vi "Main Page.vi"(8 "error in (no error)":errorcluster, 11 "Node Ptr":T1 format="%.0x") -> (0 "error out":errorcluster)   [LabVIEW 2023, in "J1939 Addon System Explorer.lvlib"]
uses:
  J1939 Addon System Explorer.lvlib
  <vilib>/NI VeriStand/Custom Device API/Custom Device Item Ref.ctl
  <vilib>/NI/NI VeriStand Hardware Resource Discovery/_Types/Filter Type.ctl
  <vilib>/NI VeriStand/Custom Device API/Custom Device File Dependency.ctl
  <vilib>/NI VeriStand/Custom Device API/Path Specification.ctl
  <vilib>/NI VeriStand/Custom Device API/Path Type.ctl
  <vilib>/NI VeriStand/Custom Device API/Custom Device Supported Target.ctl
  Addon Shared/SubVIs/Constants.vi
  <vilib>/NI VeriStand/Custom Device API/Get Item Property (Boolean).vi
  <vilib>/NI VeriStand/Custom Device API/Set Item Property (Boolean).vi
  <vilib>/NI VeriStand/Custom Device API/Set Item Property (String).vi
  <vilib>/NI VeriStand/Custom Device API/Set Item Property (Path).vi
  <vilib>/NI VeriStand/Custom Device API/Get Item Property (String).vi
  <vilib>/NI VeriStand/Custom Device API/Get Item Property (Path).vi
  <vilib>/NI VeriStand/Custom Device API/Custom Device API.lvlib
  Addon Shared/J1939 Addon Shared.lvlib
  <vilib>/NI/NI VeriStand Hardware Resource Discovery/NIVS Hardware Discovery.lvlib
panel:
  out "Version":string
  in  "RIO Browse":bool
  in  "CAN Browse":bool
  in  "Outcoming Decimation":u32=100
  in  "Incoming Decimation":u32=100
  in  "J1939 Settings 3":cluster{"Section Name":string}={"Section Name"="NI 986x Settings"}
  in  "J1939 Database Settings":cluster{"Section Name":string}={"Section Name"="J1939 Database Settings"}
  in  "RIO Device":string
  in  "Bitfile Path":path
  in  "Enable Bitfile":bool
  in  "Termination":enum16{"Off", "On"}(ring)
  in  "SHDocVw.IWebBrowser2":refnum<k7>(container)
  in  "NI 986x Settings":cluster{"Section Name":string}={"Section Name"="CAN Settings"}
  in  "CAN Port":string
  in  "Baud rate [Bd]":u32 format="%.0p"
  out "XNET Cluster":refnum<k21>
  out "XNET Database":refnum<k21>
  in  "Name":string
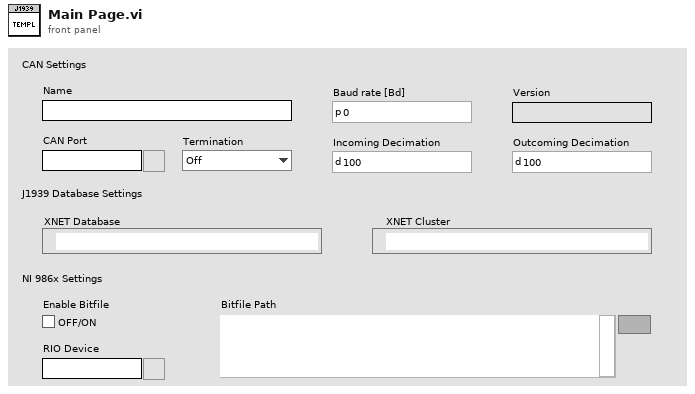
[diagram p1: front panel]
types:
  T1 = typedef "Custom Device API.lvlib/Custom Device Item Ref.ctl" = u64
  T2 = typedef "Custom Device API.lvlib/Custom Device Item Info.ctl" = cluster{"Name":string, "Is Channel":bool, "GUID":string, "Is Waveform":bool}
  T3 = typedef "J1939 Addon Shared.lvlib/XNET Settings.ctl" = cluster{"Database":refnum<k21>, "Cluster":refnum<k21>, "Port":string, "Baud rate [Bd]":u32, "Termination":u32, "Incoming Decimation":u32, "Outgoing Decimation":u32}
  T4 = typedef "NIVS Hardware Discovery.lvlib/Filter Type.ctl" = enum16{"Device Category", "Product Name", "Ethernet", "XNET", "VISA", "FPGA", "EtherCAT Master", "DAQmx", "GPIB", "Serial"}
  T5 = typedef "Custom Device API.lvlib/Custom Device File Dependency.ctl" = cluster{"Source":T6, "RT Destination":path, "ForceDownload?":bool, "SupportedTarget":T8, "Version":string}
  T6 = typedef "Custom Device API.lvlib/Path Specification.ctl" = cluster{"Path":path, "Type":T7}
  T7 = typedef "Custom Device API.lvlib/Path Type.ctl" = enum16{"Absolute", "To Base", "To Common Data Dir", "To Application Data Dir"}
  T8 = typedef "Custom Device API.lvlib/Custom Device Supported Target.ctl" = enum16{"All", "PharLap", "VxWorks", "Windows", "Linux_32_ARM", "Linux_x64", "PharLap & Windows", "PharLap & VxWorks", "VxWorks & Windows"}
  T9 = typedef "Custom Device API.lvlib/Custom Device Commands.ctl" = enum16{"Default", "Item renamed", "Shutdown", "Dynamic button pressed"}
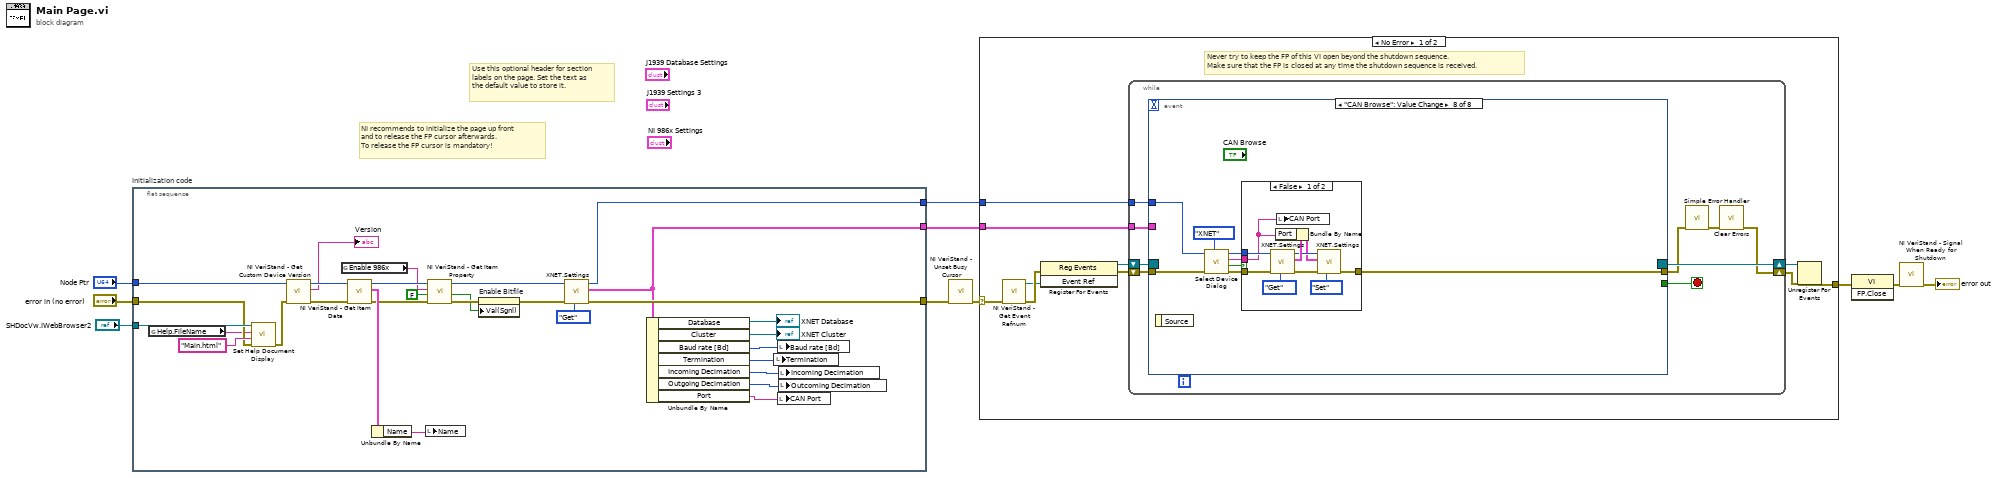
[diagram p0: block diagram]
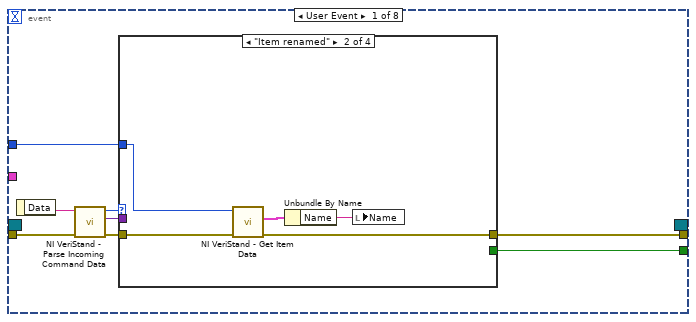
[diagram p2: hidden frame]
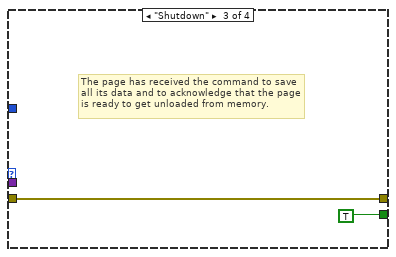
[diagram p4: hidden frame]
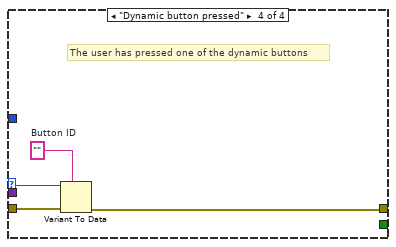
[diagram p5: hidden frame]
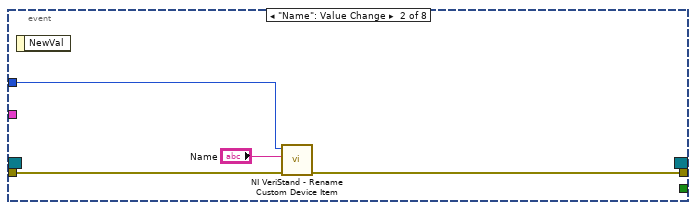
[diagram p6: hidden frame]
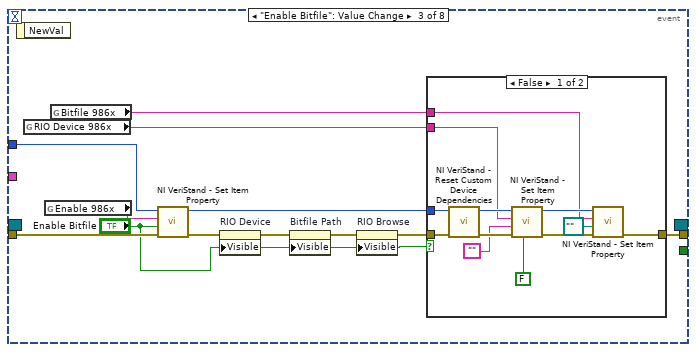
[diagram p7: hidden frame]
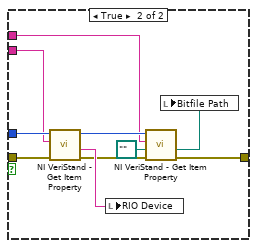
[diagram p8: hidden frame]
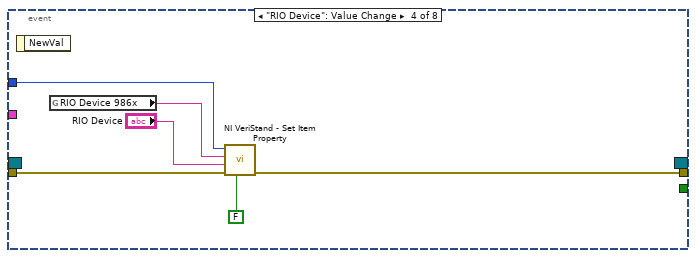
[diagram p9: hidden frame]
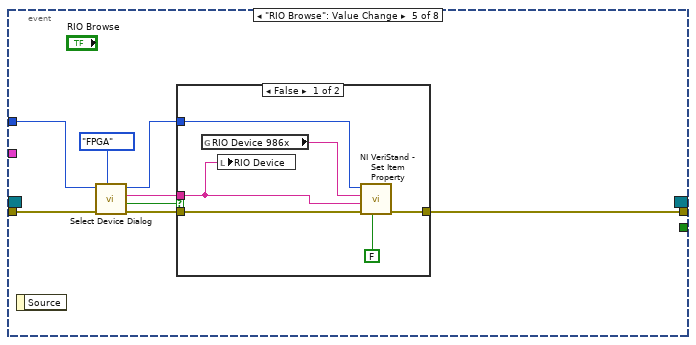
[diagram p10: hidden frame]
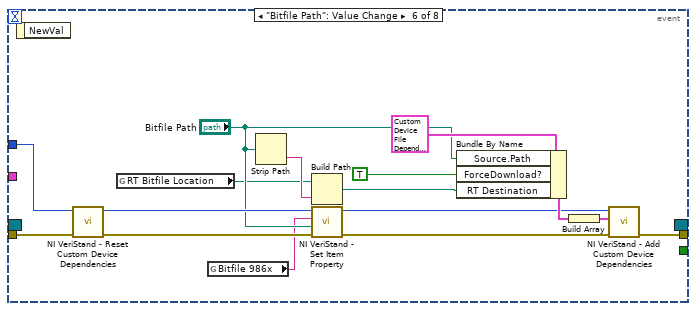
[diagram p12: hidden frame]
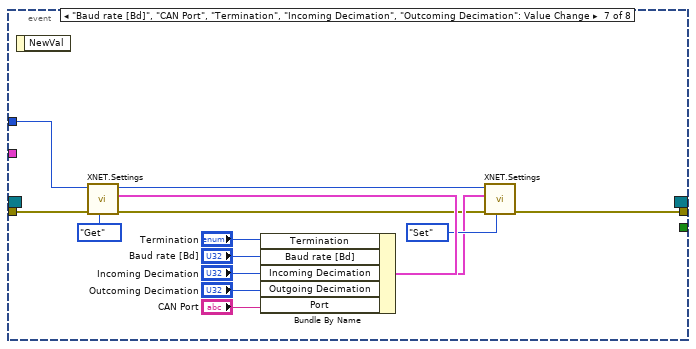
[diagram p13: hidden frame]
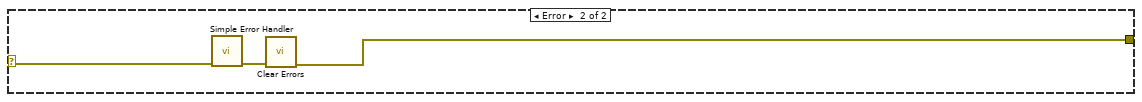
[diagram p15: hidden frame]
diagram:
  # "Use this optional header for section labels on the page. Set the text as the default value to store it."
  # "NI recommends to initialize the page up front\nand to release the FP cursor afterwards.\nTo release the FP cursor is mandatory!"
  n1 = flat-sequence "Initialization code" {
    tunnel: "error in (no error)" -> [w34]
    tunnel: "Node Ptr" -> [w13]
    tunnel: [w21] -> w6
    tunnel: [w38] -> w3
    tunnel: "SHDocVw.IWebBrowser2" -> [w35]
    tunnel: [w20] -> w1
    frame #0 {
      n2 = global read "Constants.vi" "Help.FileName"() -> (w11:string)
      n3 = call "Set Help Document Display.vi"("error in (no error)"=w34, "HTML File"="Main.html", "Main CHM File"=w11, "SHDocVw.IWebBrowser2"=w35) -> ("error out"=w16:errorcluster)  [unwired: 7 in]
      n4 = call <vilib>:"NI VeriStand - Get Custom Device Version.vi"("error in (no error)"=w16, "Device Ref in"=w13) -> ("error out"=w15:errorcluster, "Value"=→"Version":string, "Device Ref out"=w14:T1)  [unwired: 7 in]
      n5 = global read "Constants.vi" "Enable 986x"() -> (w29:string)
      n6 = call <vilib>:"NI VeriStand - Get Item Data.vi"("error in (no error)"=w15, "Item Ref in"=w14) -> ("error out"=w17:errorcluster, "Item Info"=w40:T2, "Item Ref out"=w31:T1)  [unwired: 7 out]
      n7 = Unbundle By Name(w40) -> ("Name"=w39:string)
      n8 = local write "Name"(w39) -> ()
      n9 = call-poly <vilib>:"NI VeriStand - Get Item Property.vi"("error in (no error)"=w17, "Default Value"=FALSE, "Property Name"=w29, "Item Ref in"=w31) -> ("error out"=w28:errorcluster, "Value"=w26:bool, "Item Ref out"=w30:T1)  [unwired: 4 in, 1 out]
      n10 = property on="Enable Bitfile" class="Bool (strict)"(error in=w28, "Val(Sgnl)"=w26) -> (error out=w27:errorcluster)  [unwired: 1 in, 1 out]
      n11 = call "XNET.Settings.vi"("Action"=enum8{"Get", "Set"}."Get", "error in (no error)"=w27, "Parent Ref in"=w30) -> ("error out"=w21:errorcluster, "J1939 XNET Settings"=w20:T3, "Item Ref out"=w38:T1)  [unwired: 6 in]
      n12 = Unbundle By Name(w20) -> ("Database"=→"XNET Database":refnum<k21>, "Cluster"=→"XNET Cluster":refnum<k21>, "Baud rate [Bd]"=w37:u32, "Termination"=w23:u32, "Incoming Decimation"=w24:u32, "Outgoing Decimation"=w25:u32, "Port"=w18:string)
      n13 = local write "Termination"(w23) -> ()
      n14 = local write "Baud rate [Bd]"(w37) -> ()
      n15 = local write "CAN Port"(w18) -> ()
      n16 = local write "Incoming Decimation"(w24) -> ()
      n17 = local write "Outcoming Decimation"(w25) -> ()
    }
  }
  n18 = call <vilib>:"NI VeriStand - Unset Busy Cursor.vi"("error in (no error)"=w6) -> ("error out"=w5:errorcluster)  [unwired: 10 out]
  n19 = case shown="No Error" w5 {
    selector: w5 -> [w42 w190]
    tunnel: [w47 w188] -> w10
    tunnel: w3 -> [w43 _]
    tunnel: w1 -> [w41 _]
    frame No Error {
      # "Never try to keep the FP of this VI open beyond the shutdown sequence.\nMake sure that the FP is closed at any time the shutdown sequence is received."
      n20 = call <vilib>:"NI VeriStand - Get Event Refnum.vi"("error in (no error)"=w42) -> ("error out"=w50:errorcluster, "Event Ref"=w46:refnum<user-event>)  [unwired: 9 out]
      n21 = register-events(error in=w50, w46) -> (reference out=w44:refnum<event-registration>, error out=w45:errorcluster)  [unwired: 1 in]
      n22 = while {
        tunnel: w43 -> [w55]
        shift-right: [w52] -> w48
        shift-left: w45 -> [w58]
        shift-right: [w59] -> w49
        shift-left: w44 -> [w57]
        tunnel: w41 -> [w51]
        stop <- w56 stop-if-true
        n23 = event shown="[7] \"CAN Browse\": Value Change" {
          selector: w57 -> [_ _ _ _ _ _ _ _]
          dyn-events: [_ _ _ _ _ _ _ _] -> w59
          timeout: _ -> [_ _ _ _ _ _ _ _]
          tunnel: w58 -> [w67 w83 w95 w123 w130 w154 w155 w174]
          tunnel: [w63 _ _ _ _ _ _ _] -> w56
          tunnel: [w62 w82 w90 w122 w131 w152 w159 w176] -> w54
          tunnel: w55 -> [w61 w81 w94 w121 w128 w153 w162 w175]
          tunnel: w51 -> [_ _ _ _ _ _ _ _]
          event User Event {
            n24 = event-data() -> ("Data"=w66:string)  [unwired: 1 out]
            n25 = call <vilib>:"NI VeriStand - Parse Incoming Command Data.vi"("error in (no error)"=w67, "Incoming data"=w66) -> ("error out"=w65:errorcluster, "Outgoing data"=w60:variant, "Action"=w64:T9)  [unwired: 7 out]
            n26 = case shown="\"Item renamed\"" w64 {
              tunnel: w65 -> [w68 w73 w74 w79]
              tunnel: [_ _ TRUE _] -> w63
              tunnel: [w68 w70 w74 w76] -> w62
              tunnel: w61 -> [_ w72 _ _]
              tunnel: w60 -> [_ _ _ w78]
              frame "Default", Default {
              }
              frame "Item renamed" {
                n27 = call <vilib>:"NI VeriStand - Get Item Data.vi"("error in (no error)"=w73, "Item Ref in"=w72) -> ("error out"=w70:errorcluster, "Item Info"=w71:T2)  [unwired: 8 out]
                n28 = Unbundle By Name(w71) -> ("Name"=w69:string)
                n29 = local write "Name"(w69) -> ()
              }
              frame "Shutdown" {
                # "The page has received the command to save all its data and to acknowledge that the page is ready to get unloaded from memory."
              }
              frame "Dynamic button pressed" {
                w77 = ""  # Button ID
                # "The user has pressed one of the dynamic buttons"
                n30 = Variant To Data(error in=w79, type=w77, Variant=w78) -> (error out=w76:errorcluster)  [unwired: 1 out]
              }
            }
          }
          event "Name": Value Change {
            n31 = event-data() -> ()  [unwired: 2 out]
            n32 = call <vilib>:"NI VeriStand - Rename Custom Device Item.vi"("error in (no error)"=w83, "New Name"="Name", "Item Ref in"=w81) -> ("error out"=w82:errorcluster)  [unwired: 1 in, 7 out]
          }
          event "Enable Bitfile": Value Change {
            n33 = event-data() -> ()  [unwired: 2 out]
            n34 = global read "Constants.vi" "RIO Device 986x"() -> (w88:string)
            n35 = global read "Constants.vi" "Enable 986x"() -> (w93:string)
            n36 = global read "Constants.vi" "Bitfile 986x"() -> (w87:string)
            n37 = call-poly <vilib>:"NI VeriStand - Set Item Property.vi"("error in (no error)"=w95, "Value"="Enable Bitfile", "Property Name"=w93, "Item Ref in"=w94) -> ("error out"=w91:errorcluster, "Item Ref out"=w89:T1)  [unwired: 5 in, 1 out]
            n38 = property on="RIO Device" class="Str"(error in=w91, "Visible"="Enable Bitfile") -> (error out=w92:errorcluster)  [unwired: 1 in, 1 out]
            n39 = property on="Bitfile Path" class="Path"(error in=w92, "Visible"="Enable Bitfile") -> (error out=w85:errorcluster)  [unwired: 1 in, 1 out]
            n40 = property on="RIO Browse" class="Bool"(error in=w85, "Visible"="Enable Bitfile") -> (error out=w84:errorcluster)  [unwired: 1 in, 1 out]
            n41 = case shown="False" "Enable Bitfile" {
              tunnel: w84 -> [w107 w117]
              tunnel: [w103 w112] -> w90
              tunnel: w89 -> [w106 w116]
              tunnel: w88 -> [w100 w115]
              tunnel: w87 -> [w99 w109]
              frame False {
                n42 = call <vilib>:"NI VeriStand - Reset Custom Device Dependencies.vi"("error in (no error)"=w107, "Device Ref in"=w106) -> ("error out"=w104:errorcluster, "Device Ref out"=w102:T1)  [unwired: 8 in]
                n43 = call-poly <vilib>:"NI VeriStand - Set Item Property.vi"("Binary String (T)"=FALSE, "error in (no error)"=w104, "Value"="", "Property Name"=w100, "Item Ref in"=w102) -> ("error out"=w105:errorcluster, "Item Ref out"=w101:T1)  [unwired: 4 in, 1 out]
                n44 = call-poly <vilib>:"NI VeriStand - Set Item Property.vi"("error in (no error)"=w105, "Value"=path "", "Property Name"=w99, "Item Ref in"=w101) -> ("error out"=w103:errorcluster)  [unwired: 5 in, 2 out]
              }
              frame True {
                n45 = call-poly <vilib>:"NI VeriStand - Get Item Property.vi"("error in (no error)"=w117, "Property Name"=w115, "Item Ref in"=w116) -> ("error out"=w113:errorcluster, "Value"=w114:string, "Item Ref out"=w110:T1)  [unwired: 5 in, 1 out]
                n46 = local write "RIO Device"(w114) -> ()
                n47 = call-poly <vilib>:"NI VeriStand - Get Item Property.vi"("error in (no error)"=w113, "Default Value"=path "", "Property Name"=w109, "Item Ref in"=w110) -> ("error out"=w112:errorcluster, "Value"=w108:path)  [unwired: 4 in, 2 out]
                n48 = local write "Bitfile Path"(w108) -> ()
              }
            }
          }
          event "RIO Device": Value Change {
            n49 = event-data() -> ()  [unwired: 2 out]
            n50 = global read "Constants.vi" "RIO Device 986x"() -> (w120:string)
            n51 = call-poly <vilib>:"NI VeriStand - Set Item Property.vi"("Binary String (T)"=FALSE, "error in (no error)"=w123, "Value"="RIO Device", "Property Name"=w120, "Item Ref in"=w121) -> ("error out"=w122:errorcluster)  [unwired: 4 in, 2 out]
          }
          event "RIO Browse": Value Change {
            n52 = event-data() -> ()  [unwired: 2 out]
            n53 = call <vilib>:"Select Device Dialog.vi"("Filter Type"=Filter_Type."FPGA", "error in (no error)"=w130, "Item Ref in"=w128) -> ("error out"=w129:errorcluster, "Cancelled?"=w126:bool, "Selected Alias"=w125:string, "Item Ref out"=w127:T1)  [unwired: 5 in]
            n54 = case shown="False" w126 {
              tunnel: w129 -> [w137 w138]
              tunnel: [w136 w138] -> w131
              tunnel: w127 -> [w135 _]
              tunnel: w125 -> [w132 _]
              frame False {
                n55 = global read "Constants.vi" "RIO Device 986x"() -> (w134:string)
                n56 = local write "RIO Device"(w132) -> ()
                n57 = call-poly <vilib>:"NI VeriStand - Set Item Property.vi"("Binary String (T)"=FALSE, "error in (no error)"=w137, "Value"=w132, "Property Name"=w134, "Item Ref in"=w135) -> ("error out"=w136:errorcluster)  [unwired: 4 in, 2 out]
              }
              frame True {
              }
            }
          }
          event "Bitfile Path": Value Change {
            n58 = event-data() -> ()  [unwired: 2 out]
            n59 = call <vilib>:"NI VeriStand - Reset Custom Device Dependencies.vi"("error in (no error)"=w154, "Device Ref in"=w153) -> ("error out"=w145:errorcluster, "Device Ref out"=w142:T1)  [unwired: 8 in]
            n60 = global read "Constants.vi" "RT Bitfile Location"() -> (w139:path)
            n61 = global read "Constants.vi" "Bitfile 986x"() -> (w140:string)
            n62 = Strip Path(path="Bitfile Path") -> (name=w147:string)  [unwired: 1 out]
            n63 = Build Path(base path=w139, name or relative path=w147) -> (appended path=w146:path)
            n64 = call-poly <vilib>:"NI VeriStand - Set Item Property.vi"("error in (no error)"=w145, "Value"="Bitfile Path", "Property Name"=w140, "Item Ref in"=w142) -> ("error out"=w144:errorcluster, "Item Ref out"=w143:T1)  [unwired: 5 in, 1 out]
            n65 = Bundle By Name(cluster=T5 {"Source"={"Path"=path "", "Type"=enum."Absolute"}, "RT Destination"=path "", "ForceDownload?"=FALSE, "SupportedTarget"=enum."PharLap", "Version"=""} ("Dependency"), "Source.Path"="Bitfile Path", "ForceDownload?"=TRUE, "RT Destination"=w146) -> (w150:T5)
            n66 = Build Array(w150) -> (w149:T5[])
            n67 = call <vilib>:"NI VeriStand - Add Custom Device Dependencies.vi"("error in (no error)"=w144, "Dependencies"=w149, "Device Ref in"=w143) -> ("error out"=w152:errorcluster)  [unwired: 7 in, 1 out]
          }
          event "Baud rate [Bd]", "CAN Port", "Termination", "Incoming Decimation", "Outcoming Decimation": Value Change {
            n68 = event-data() -> ()  [unwired: 2 out]
            n69 = call "XNET.Settings.vi"("Action"=enum8{"Get", "Set"}."Get", "error in (no error)"=w155, "Parent Ref in"=w162) -> ("error out"=w157:errorcluster, "J1939 XNET Settings"=w163:T3, "Item Ref out"=w160:T1)  [unwired: 6 in]
            n70 = Bundle By Name(cluster=w163, "Termination"="Termination", "Baud rate [Bd]"="Baud rate [Bd]", "Incoming Decimation"="Incoming Decimation", "Outgoing Decimation"="Outcoming Decimation", "Port"="CAN Port") -> (w158:T3)
            n71 = call "XNET.Settings.vi"("Action"=enum8{"Get", "Set"}."Set", "error in (no error)"=w157, "J1939 XNET Settings"=w158, "Parent Ref in"=w160) -> ("error out"=w159:errorcluster)  [unwired: 5 in, 2 out]
          }
          event "CAN Browse": Value Change {
            n72 = event-data() -> ()  [unwired: 2 out]
            n73 = call <vilib>:"Select Device Dialog.vi"("Filter Type"=Filter_Type."XNET", "error in (no error)"=w174, "Item Ref in"=w175) -> ("error out"=w172:errorcluster, "Cancelled?"=w171:bool, "Selected Alias"=w170:string, "Item Ref out"=w173:T1)  [unwired: 5 in]
            n74 = case shown="False" w171 {
              tunnel: w173 -> [w184 _]
              tunnel: [w181 w187] -> w176
              tunnel: w172 -> [w178 w187]
              tunnel: w170 -> [w177 _]
              frame False {
                n75 = call "XNET.Settings.vi"("Action"=enum8{"Get", "Set"}."Get", "error in (no error)"=w178, "Parent Ref in"=w184) -> ("error out"=w179:errorcluster, "J1939 XNET Settings"=w185:T3, "Item Ref out"=w182:T1)  [unwired: 6 in]
                n76 = Bundle By Name(cluster=w185, "Port"=w177) -> (w180:T3)
                n77 = local write "CAN Port"(w177) -> ()
                n78 = call "XNET.Settings.vi"("Action"=enum8{"Get", "Set"}."Set", "error in (no error)"=w179, "J1939 XNET Settings"=w180, "Parent Ref in"=w182) -> ("error out"=w181:errorcluster)  [unwired: 5 in, 2 out]
              }
              frame True {
              }
            }
          }
        }
        n79 = call <vilib>:"Simple Error Handler.vi"("error in (no error)"=w54) -> ("error out"=w53:errorcluster)  [unwired: 1 in, 7 out]
        n80 = call <vilib>:"Clear Errors.vi"("error in (no error)"=w53) -> ("error out"=w52:errorcluster)  [unwired: 1 in, 5 out]
      }
      n81 = Unregister For Events(event registration refnum=w49, error in=w48) -> (error out=w47:errorcluster)
    }
    frame Error {
      n82 = call <vilib>:"Simple Error Handler.vi"("error in (no error)"=w190) -> ("error out"=w189:errorcluster)  [unwired: 1 in, 7 out]
      n83 = call <vilib>:"Clear Errors.vi"("error in (no error)"=w189) -> ("error out"=w188:errorcluster)  [unwired: 1 in, 5 out]
    }
  }
  n84 = invoke class="VI" method="FP.Close"(error in=w10) -> (error out=w9:errorcluster)  [unwired: 2 in, 2 out]
  n85 = call <vilib>:"NI VeriStand - Signal When Ready for Shutdown.vi"("error in (no error)"=w9) -> ("error out"=→"error out":errorcluster)  [unwired: 10 out]
